vi "Main.vi"() -> ()   [LabVIEW 2014]
panel:
  out "loop 2":dbl
  in  "Event Control Switch":bool
  out "loop 1":dbl
  in  "App Stop":bool
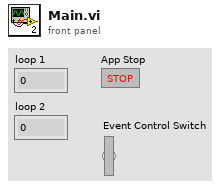
[diagram p1: front panel]
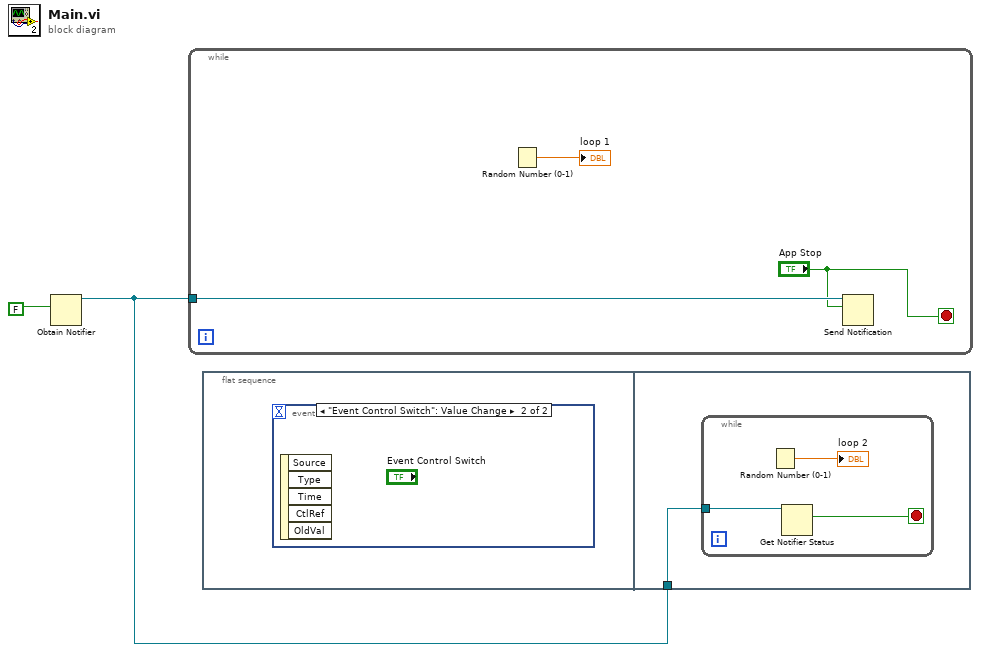
[diagram p0: block diagram]
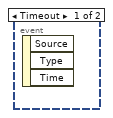
[diagram p2: hidden frame]
diagram:
  n1 = Obtain Notifier(notification data type=FALSE) -> (notifier out=w1:refnum<notifier>)  [unwired: 3 in, 2 out]
  n2 = while {
    tunnel: w1 -> [w5]
    stop <- "App Stop" stop-if-true
    n3 = Random Number (0-1)() -> (number: 0 to 1=→"loop 1":dbl)
    n4 = Send Notification(notification="App Stop", notifier=w5) -> ()  [unwired: 1 in, 2 out]
  }
  n5 = flat-sequence {
    tunnel: w1 -> [w6]
    frame #0 {
      n6 = event shown="[1] \"Event Control Switch\": Value Change" {
        selector: _ -> [_ _]
        dyn-events: _ -> [_ _]
        timeout: _ -> [_ _]
        event Timeout {
          n7 = event-data() -> ()  [unwired: 1 in, 3 out]
        }
        event "Event Control Switch": Value Change {
          n8 = event-data() -> ()  [unwired: 1 in, 5 out]
        }
      }
    }
    frame #1 {
      n9 = while {
        tunnel: w6 -> [w8]
        stop <- w7 stop-if-true
        n10 = Random Number (0-1)() -> (number: 0 to 1=→"loop 2":dbl)
        n11 = Get Notifier Status(notifier=w8) -> (current notification=w7:bool)  [unwired: 1 in, 4 out]
      }
    }
  }
